vi "Lab Panel V6.00.vi"() -> ()   [LabVIEW 2017] (continued)
                        n3252 = Unbundle By Name(w5931) -> ("1 (TL) cal"=w5926:dbl, "1 (TN) cal"=w5925:dbl, "2 (TL) cal"=w5924:dbl, "2 (TN) cal"=w5923:dbl)  [unwired: 6 out]
                        n3253 = local write "TEMP LA03"(w5920) -> ()
                        n3254 = Multiply(x=w5919, y=w5926) -> (x*y=w5912:dbl)
                        n3255 = Multiply(x=w5918, y=w5925) -> (x*y=w5911:dbl)
                        n3256 = Multiply(x=w5917, y=w5924) -> (x*y=w5908:dbl)
                        n3257 = Multiply(x=w5916, y=w5923) -> (x*y=w5907:dbl)
                        n3258 = case shown="True" w5903 {
                          tunnel: w5908 -> [w5933 w5938]
                          tunnel: w5913 -> [_ w5936]
                          tunnel: [w5933 w5937] -> w5906
                          tunnel: w5907 -> [w5932 w5935]
                          tunnel: [w5932 w5934] -> w5905
                          frame False {
                          }
                          frame True {
                            n3259 = Multiply(x=w5936, y=w5935) -> (x*y=w5934:dbl)
                            n3260 = Multiply(x=w5936, y=w5938) -> (x*y=w5937:dbl)
                          }
                        }
                        n3261 = case shown="True" w5904 {
                          tunnel: w5912 -> [w5940 w5945]
                          tunnel: w5913 -> [_ w5943]
                          tunnel: [w5940 w5944] -> w5910
                          tunnel: w5911 -> [w5939 w5942]
                          tunnel: [w5939 w5941] -> w5909
                          frame False {
                          }
                          frame True {
                            n3262 = Multiply(x=w5943, y=w5942) -> (x*y=w5941:dbl)
                            n3263 = Multiply(x=w5943, y=w5945) -> (x*y=w5944:dbl)
                          }
                        }
                        n3264 = local read "SIG LAB03-2"() -> (w5928:T2)
                        n3265 = local read "SIG LAB03-1"() -> (w5930:T2)
                        n3266 = Bundle By Name(cluster=w5928, "Tmp Live"=w5906, "Tmp Neut"=w5905) -> (w5927:T2)
                        n3267 = Bundle By Name(cluster=w5930, "Tmp Live"=w5910, "Tmp Neut"=w5909) -> (w5929:T2)
                        n3268 = local write "SIG LAB03-2"(w5927) -> ()
                        n3269 = local write "SIG LAB03-1"(w5929) -> ()
                      }
                      frame #4 {
                        n3270 = case shown="False" w5960 {
                          tunnel: [w5991 w5992] -> w5976
                          tunnel: w5959 -> [_ w5992]
                          frame False {
                            n3271 = local read "CAL LAB04"() -> (w5991:T15)
                          }
                          frame True {
                          }
                        }
                        n3272 = local read "LAB04 TEMP"() -> (w5966:T13)
                        n3273 = local read "TEMP LA04"() -> (w5967:T10)
                        n3274 = call "sub vi - temperature delay v4.vi"("2-run"=w5948, "1-run"=w5949, "temp values IN"=w5967, "temp signals"=w5966) -> ("T2-N"=w5961:dbl, "T2-L"=w5962:dbl, "T1-N"=w5963:dbl, "T1-L"=w5964:dbl, "temp values OUT"=w5965:T47)  [unwired: 3 in]
                        n3275 = Unbundle By Name(w5976) -> ("1 (TL) cal"=w5971:dbl, "1 (TN) cal"=w5970:dbl, "2 (TL) cal"=w5969:dbl, "2 (TN) cal"=w5968:dbl)  [unwired: 6 out]
                        n3276 = local write "TEMP LA04"(w5965) -> ()
                        n3277 = Multiply(x=w5964, y=w5971) -> (x*y=w5957:dbl)
                        n3278 = Multiply(x=w5963, y=w5970) -> (x*y=w5956:dbl)
                        n3279 = Multiply(x=w5962, y=w5969) -> (x*y=w5953:dbl)
                        n3280 = Multiply(x=w5961, y=w5968) -> (x*y=w5952:dbl)
                        n3281 = case shown="True" w5948 {
                          tunnel: w5953 -> [w5978 w5983]
                          tunnel: w5958 -> [_ w5981]
                          tunnel: [w5978 w5982] -> w5951
                          tunnel: w5952 -> [w5977 w5980]
                          tunnel: [w5977 w5979] -> w5950
                          frame False {
                          }
                          frame True {
                            n3282 = Multiply(x=w5981, y=w5980) -> (x*y=w5979:dbl)
                            n3283 = Multiply(x=w5981, y=w5983) -> (x*y=w5982:dbl)
                          }
                        }
                        n3284 = case shown="True" w5949 {
                          tunnel: w5957 -> [w5985 w5990]
                          tunnel: w5958 -> [_ w5988]
                          tunnel: [w5985 w5989] -> w5955
                          tunnel: w5956 -> [w5984 w5987]
                          tunnel: [w5984 w5986] -> w5954
                          frame False {
                          }
                          frame True {
                            n3285 = Multiply(x=w5988, y=w5987) -> (x*y=w5986:dbl)
                            n3286 = Multiply(x=w5988, y=w5990) -> (x*y=w5989:dbl)
                          }
                        }
                        n3287 = local read "SIG LAB04-2"() -> (w5973:T2)
                        n3288 = local read "SIG LAB04-1"() -> (w5975:T2)
                        n3289 = Bundle By Name(cluster=w5973, "Tmp Live"=w5951, "Tmp Neut"=w5950) -> (w5972:T2)
                        n3290 = Bundle By Name(cluster=w5975, "Tmp Live"=w5955, "Tmp Neut"=w5954) -> (w5974:T2)
                        n3291 = local write "SIG LAB04-2"(w5972) -> ()
                        n3292 = local write "SIG LAB04-1"(w5974) -> ()
                      }
                      frame #5 {
                        n3293 = case shown="False" w6005 {
                          tunnel: [w6036 w6037] -> w6021
                          tunnel: w6004 -> [_ w6037]
                          frame False {
                            n3294 = local read "CAL LAB05"() -> (w6036:T15)
                          }
                          frame True {
                          }
                        }
                        n3295 = local read "LAB05 TEMP"() -> (w6011:T13)
                        n3296 = local read "TEMP LA05"() -> (w6012:T10)
                        n3297 = call "sub vi - temperature delay v4.vi"("2-run"=w5993, "1-run"=w5994, "temp values IN"=w6012, "temp signals"=w6011) -> ("T2-N"=w6007:dbl, "T2-L"=w6008:dbl, "T1-N"=w6009:dbl, "T1-L"=w6010:dbl, "temp values OUT"=w6006:T47)  [unwired: 3 in]
                        n3298 = local write "TEMP LA05"(w6006) -> ()
                        n3299 = Unbundle By Name(w6021) -> ("1 (TL) cal"=w6013:dbl, "1 (TN) cal"=w6016:dbl, "2 (TL) cal"=w6015:dbl, "2 (TN) cal"=w6014:dbl)  [unwired: 6 out]
                        n3300 = Multiply(x=w6010, y=w6013) -> (x*y=w6002:dbl)
                        n3301 = Multiply(x=w6009, y=w6016) -> (x*y=w6001:dbl)
                        n3302 = Multiply(x=w6008, y=w6015) -> (x*y=w5998:dbl)
                        n3303 = Multiply(x=w6007, y=w6014) -> (x*y=w5997:dbl)
                        n3304 = case shown="True" w5993 {
                          tunnel: w5998 -> [w6023 w6028]
                          tunnel: w6003 -> [_ w6026]
                          tunnel: [w6023 w6027] -> w5996
                          tunnel: w5997 -> [w6022 w6025]
                          tunnel: [w6022 w6024] -> w5995
                          frame False {
                          }
                          frame True {
                            n3305 = Multiply(x=w6026, y=w6025) -> (x*y=w6024:dbl)
                            n3306 = Multiply(x=w6026, y=w6028) -> (x*y=w6027:dbl)
                          }
                        }
                        n3307 = case shown="True" w5994 {
                          tunnel: w6002 -> [w6030 w6035]
                          tunnel: w6003 -> [_ w6033]
                          tunnel: [w6030 w6034] -> w6000
                          tunnel: w6001 -> [w6029 w6032]
                          tunnel: [w6029 w6031] -> w5999
                          frame False {
                          }
                          frame True {
                            n3308 = Multiply(x=w6033, y=w6032) -> (x*y=w6031:dbl)
                            n3309 = Multiply(x=w6033, y=w6035) -> (x*y=w6034:dbl)
                          }
                        }
                        n3310 = local read "SIG LAB05-1"() -> (w6020:T2)
                        n3311 = Bundle By Name(cluster=w6020, "Tmp Live"=w6000, "Tmp Neut"=w5999) -> (w6019:T2)
                        n3312 = local read "SIG LAB05-2"() -> (w6018:T2)
                        n3313 = Bundle By Name(cluster=w6018, "Tmp Live"=w5996, "Tmp Neut"=w5995) -> (w6017:T2)
                        n3314 = local write "SIG LAB05-1"(w6019) -> ()
                        n3315 = local write "SIG LAB05-2"(w6017) -> ()
                      }
                      frame #6 {
                        w6138 = 150.0
                        # "check for thermocouple error, output >150 deg??"
                        n3316 = local read "SIG LAB01-2"() -> (w6147:T2)
                        n3317 = local read "SIG LAB01-1"() -> (w6148:T2)
                        n3318 = local read "SIG LAB04-1"() -> (w6141:T2)
                        n3319 = local read "SIG LAB04-2"() -> (w6142:T2)
                        n3320 = Unbundle By Name(w6148) -> ("Tmp Live"=w6076:dbl, "Tmp Neut"=w6074:dbl)
                        n3321 = Unbundle(w6142) -> ("Tmp Live"=w6052:dbl, "Tmp Neut"=w6051:dbl)  [unwired: 3 out]
                        n3322 = Unbundle(w6147) -> ("Tmp Live"=w6073:dbl, "Tmp Neut"=w6071:dbl)  [unwired: 3 out]
                        n3323 = Unbundle(w6141) -> ("Tmp Live"=w6053:dbl, "Tmp Neut"=w6046:dbl)  [unwired: 3 out]
                        n3324 = Absolute Value(x=w6053) -> (abs(x)=w6047:dbl)
                        n3325 = Absolute Value(x=w6046) -> (abs(x)=w6048:dbl)
                        n3326 = Absolute Value(x=w6052) -> (abs(x)=w6050:dbl)
                        n3327 = Absolute Value(x=w6051) -> (abs(x)=w6049:dbl)
                        n3328 = Absolute Value(x=w6073) -> (abs(x)=w6072:dbl)
                        n3329 = Absolute Value(x=w6071) -> (abs(x)=w6070:dbl)
                        n3330 = Absolute Value(x=w6074) -> (abs(x)=w6075:dbl)
                        n3331 = Absolute Value(x=w6076) -> (abs(x)=w6077:dbl)
                        n3332 = Greater?(x=w6049, y=w6138) -> (0:w6114:bool)
                        "LA04-2 (TN)" <- w6114
                        n3333 = Greater?(x=w6070, y=w6138) -> (0:w6126:bool)
                        "LA01-2 (TN)" <- w6126
                        n3334 = Greater?(x=w6050, y=w6138) -> (0:w6115:bool)
                        "LA04-2 (TL)" <- w6115
                        n3335 = Greater?(x=w6072, y=w6138) -> (0:w6127:bool)
                        "LA01-2 (TL)" <- w6127
                        n3336 = Greater?(x=w6048, y=w6138) -> (0:w6116:bool)
                        "LA04-1 (TN)" <- w6116
                        n3337 = Greater?(x=w6075, y=w6138) -> (0:w6137:bool)
                        "LA01-1 (TN)" <- w6137
                        n3338 = Greater?(x=w6047, y=w6138) -> (0:w6117:bool)
                        "LA04-1 (TL)" <- w6117
                        n3339 = Greater?(x=w6077, y=w6138) -> (0:w6136:bool)
                        "LA01-1 (TL)" <- w6136
                        n3340 = Or(x=w6137, y=w6136) -> (x .or. y?=w6135:bool)
                        n3341 = Or(x=w6114, y=w6115) -> (x .or. y?=w6125:bool)
                        n3342 = Or(x=w6127, y=w6126) -> (x .or. y?=w6131:bool)
                        n3343 = Or(x=w6116, y=w6117) -> (x .or. y?=w6121:bool)
                        n3344 = Select(t=u32 16711680, s=w6135, f=u32 13816530) -> (s? t:f=w6132:u32)
                        n3345 = Select(t=u32 16711680, s=w6125, f=u32 13816530) -> (s? t:f=w6122:u32)
                        n3346 = Select(t=u32 16711680, s=w6131, f=u32 13816530) -> (s? t:f=w6128:u32)
                        n3347 = Select(t=u32 16711680, s=w6121, f=u32 13816530) -> (s? t:f=w6118:u32)
                        n3348 = property on="SIG LAB01-1" class="Clust (strict)"("Color"=w6132) -> ()  [unwired: 2 in, 2 out]
                        n3349 = property on="SIG LAB01-2" class="Clust (strict)"("Color"=w6128) -> ()  [unwired: 2 in, 2 out]
                        n3350 = property on="SIG LAB04-2" class="Clust (strict)"("Color"=w6122) -> ()  [unwired: 2 in, 2 out]
                        n3351 = property on="SIG LAB04-1" class="Clust (strict)"("Color"=w6118) -> ()  [unwired: 2 in, 2 out]
                        n3352 = local read "SIG LAB02-1"() -> (w6145:T2)
                        n3353 = local read "SIG LAB02-2"() -> (w6146:T2)
                        n3354 = local read "SIG LAB05-2"() -> (w6139:T2)
                        n3355 = local read "SIG LAB05-1"() -> (w6140:T2)
                        n3356 = Unbundle(w6146) -> ("Tmp Live"=w6065:dbl, "Tmp Neut"=w6063:dbl)  [unwired: 3 out]
                        n3357 = Unbundle(w6145) -> ("Tmp Live"=w6069:dbl, "Tmp Neut"=w6068:dbl)  [unwired: 3 out]
                        n3358 = Unbundle(w6139) -> ("Tmp Live"=w6041:dbl, "Tmp Neut"=w6039:dbl)  [unwired: 3 out]
                        n3359 = Unbundle(w6140) -> ("Tmp Live"=w6045:dbl, "Tmp Neut"=w6043:dbl)  [unwired: 3 out]
                        n3360 = Absolute Value(x=w6065) -> (abs(x)=w6064:dbl)
                        n3361 = Absolute Value(x=w6063) -> (abs(x)=w6062:dbl)
                        n3362 = Absolute Value(x=w6068) -> (abs(x)=w6066:dbl)
                        n3363 = Absolute Value(x=w6069) -> (abs(x)=w6067:dbl)
                        n3364 = Absolute Value(x=w6041) -> (abs(x)=w6040:dbl)
                        n3365 = Absolute Value(x=w6039) -> (abs(x)=w6038:dbl)
                        n3366 = Absolute Value(x=w6045) -> (abs(x)=w6044:dbl)
                        n3367 = Absolute Value(x=w6043) -> (abs(x)=w6042:dbl)
                        n3368 = Greater?(x=w6062, y=w6138) -> (0:w6090:bool)
                        "LA02-2 (TN)" <- w6090
                        n3369 = Greater?(x=w6064, y=w6138) -> (0:w6091:bool)
                        "LA02-2 (TL)" <- w6091
                        n3370 = Greater?(x=w6066, y=w6138) -> (0:w6093:bool)
                        "LA02-1 (TN)" <- w6093
                        n3371 = Greater?(x=w6067, y=w6138) -> (0:w6092:bool)
                        "LA02-1 (TL)" <- w6092
                        n3372 = Greater?(x=w6038, y=w6138) -> (0:w6102:bool)
                        "LA05-2 (TN)" <- w6102
                        n3373 = Greater?(x=w6040, y=w6138) -> (0:w6103:bool)
                        "LA05-2 (TL)" <- w6103
                        n3374 = Greater?(x=w6042, y=w6138) -> (0:w6104:bool)
                        "LA05-1 (TN)" <- w6104
                        n3375 = Greater?(x=w6044, y=w6138) -> (0:w6105:bool)
                        "LA05-1 (TL)" <- w6105
                        n3376 = Or(x=w6093, y=w6092) -> (x .or. y?=w6101:bool)
                        n3377 = Or(x=w6091, y=w6090) -> (x .or. y?=w6097:bool)
                        n3378 = Or(x=w6105, y=w6104) -> (x .or. y?=w6113:bool)
                        n3379 = Or(x=w6103, y=w6102) -> (x .or. y?=w6109:bool)
                        n3380 = Select(t=u32 16711680, s=w6101, f=u32 13816530) -> (s? t:f=w6098:u32)
                        n3381 = Select(t=u32 16711680, s=w6097, f=u32 13816530) -> (s? t:f=w6094:u32)
                        n3382 = Select(t=u32 16711680, s=w6113, f=u32 13816530) -> (s? t:f=w6110:u32)
                        n3383 = local read "SIG LAB03-1"() -> (w6143:T2)
                        n3384 = Select(t=u32 16711680, s=w6109, f=u32 13816530) -> (s? t:f=w6106:u32)
                        n3385 = property on="SIG LAB02-1" class="Clust (strict)"("Color"=w6098) -> ()  [unwired: 2 in, 2 out]
                        n3386 = property on="SIG LAB02-2" class="Clust (strict)"("Color"=w6094) -> ()  [unwired: 2 in, 2 out]
                        n3387 = local read "SIG LAB03-2"() -> (w6144:T2)
                        n3388 = property on="SIG LAB05-1" class="Clust (strict)"("Color"=w6110) -> ()  [unwired: 2 in, 2 out]
                        n3389 = property on="SIG LAB05-2" class="Clust (strict)"("Color"=w6106) -> ()  [unwired: 2 in, 2 out]
                        n3390 = Unbundle(w6144) -> ("Tmp Live"=w6057:dbl, "Tmp Neut"=w6055:dbl)  [unwired: 3 out]
                        n3391 = Unbundle(w6143) -> ("Tmp Live"=w6061:dbl, "Tmp Neut"=w6059:dbl)  [unwired: 3 out]
                        n3392 = Absolute Value(x=w6057) -> (abs(x)=w6056:dbl)
                        n3393 = Absolute Value(x=w6055) -> (abs(x)=w6054:dbl)
                        n3394 = Absolute Value(x=w6061) -> (abs(x)=w6060:dbl)
                        n3395 = Absolute Value(x=w6059) -> (abs(x)=w6058:dbl)
                        n3396 = Greater?(x=w6054, y=w6138) -> (0:w6078:bool)
                        "LA03-2 (TN)" <- w6078
                        n3397 = Greater?(x=w6056, y=w6138) -> (0:w6079:bool)
                        "LA03-2 (TL)" <- w6079
                        n3398 = Greater?(x=w6058, y=w6138) -> (0:w6081:bool)
                        "LA03-1 (TN)" <- w6081
                        n3399 = Greater?(x=w6060, y=w6138) -> (0:w6080:bool)
                        "LA03-1 (TL)" <- w6080
                        n3400 = Or(x=w6081, y=w6080) -> (x .or. y?=w6089:bool)
                        n3401 = Or(x=w6079, y=w6078) -> (x .or. y?=w6085:bool)
                        n3402 = Select(t=u32 16711680, s=w6089, f=u32 13816530) -> (s? t:f=w6086:u32)
                        n3403 = Select(t=u32 16711680, s=w6085, f=u32 13816530) -> (s? t:f=w6082:u32)
                        n3404 = property on="SIG LAB03-1" class="Clust (strict)"("Color"=w6086) -> ()  [unwired: 2 in, 2 out]
                        n3405 = property on="SIG LAB03-2" class="Clust (strict)"("Color"=w6082) -> ()  [unwired: 2 in, 2 out]
                      }
                    }
                  }
                }
              }
            }
          }
          frame #22 {
            # "SAVE ON AMPS VALUES FOR REPORT FILE"
            # "write data to display panel"
            n3406 = global write "Global display 1.vi" "TEST 5-2"(w6184) -> ()
            n3407 = global write "Global display 1.vi" "TEST 4-2"(w6186) -> ()
            n3408 = global write "Global display 1.vi" "TEST 1-2"(w6192) -> ()
            n3409 = global write "Global display 1.vi" "TEST 3-1"(w6189) -> ()
            n3410 = global write "Global display 1.vi" "TEST 5-1"(w6185) -> ()
            n3411 = global write "Global display 1.vi" "TEST 1-1"(w6193) -> ()
            n3412 = global write "Global display 1.vi" "TEST 3-2"(w6188) -> ()
            n3413 = global write "Global display 1.vi" "TEST 4-1"(w6187) -> ()
            n3414 = global write "Global display 1.vi" "TEST 2-2"(w6190) -> ()
            n3415 = global write "Global display 1.vi" "TEST 2-1"(w6191) -> ()
            n3416 = global read "Global display 3.vi" "log 1-1"() -> (→"LOG LAB01-1":string)
            n3417 = global read "Global display 3.vi" "log 3-1"() -> (→"LOG LAB03-1":string)
            n3418 = global read "Global display 3.vi" "log 1-2"() -> (→"LOG LAB01-2":string)
            n3419 = property on="Tab Control 2" class="TabCtl (strict)"() -> ("Pages"=w6183:refnum<vi>[])  [unwired: 2 in, 2 out]
            n3420 = global read "Global display 3.vi" "log 2-1"() -> (→"LOG LAB02-1":string)
            n3421 = global read "Global display 3.vi" "log 2-2"() -> (→"LOG LAB02-2":string)
            n3422 = global read "Global display 3.vi" "log 4-2"() -> (→"LOG LAB04-2":string)
            n3423 = global read "Global display 3.vi" "log 5-2"() -> (→"LOG LAB05-2":string)
            n3424 = global read "Global display 3.vi" "log 5-1"() -> (→"LOG LAB05-1":string)
            n3425 = global read "Global display 3.vi" "log 4-1"() -> (→"LOG LAB04-1":string)
            n3426 = global read "Global display 3.vi" "log 3-2"() -> (→"LOG LAB03-2":string)
            n3427 = Index Array(array=w6183, index=8) -> (element=w6181:refnum<vi>)
            n3428 = property class="Page"(reference=w6181) -> ("PageVis"=w6180:bool)  [unwired: 1 in, 2 out]
            n3429 = local read "DISP LAB03-1"() -> (w6219:T4)
            n3430 = local read "DISP LAB04-2"() -> (w6216:T4)
            n3431 = local read "DISP LAB05-1"() -> (w6215:T4)
            n3432 = local read "DISP LAB01-2"() -> (w6222:T4)
            n3433 = local read "DISP LAB02-1"() -> (w6221:T4)
            n3434 = local read "DISP LAB02-2"() -> (w6220:T4)
            n3435 = local read "DISP LAB04-1"() -> (w6217:T4)
            n3436 = local read "DISP LAB05-2"() -> (w6214:T4)
            n3437 = local read "DISP LAB01-1"() -> (w6223:T4)
            n3438 = local read "DISP LAB03-2"() -> (w6218:T4)
            n3439 = global write "Global display 3.vi" "admin"(w6180) -> ()
            n3440 = local read "O/I  LAB05-2"() -> (w6234:bool)
            n3441 = local read "O/I  LAB05-1"() -> (w6235:bool)
            n3442 = local read "O/I  LAB03-2"() -> (w6238:bool)
            n3443 = local read "O/I  LAB04-2"() -> (w6236:bool)
            n3444 = local read "O/I  LAB04-1"() -> (w6237:bool)
            n3445 = local read "O/I  LAB03-1"() -> (w6239:bool)
            n3446 = local read "O/I  LAB01-2"() -> (w6242:bool)
            n3447 = local read "O/I  LAB01-1"() -> (w6243:bool)
            n3448 = local read "O/I  LAB02-1"() -> (w6241:bool)
            n3449 = local read "O/I  LAB02-2"() -> (w6240:bool)
            n3450 = global write "Global display 1.vi" "5-2 O/F"(w6234) -> ()
            n3451 = global write "Global display 1.vi" "5-1 O/F"(w6235) -> ()
            n3452 = global write "Global display 1.vi" "4-1 O/F"(w6237) -> ()
            n3453 = global write "Global display 1.vi" "4-2 O/F"(w6236) -> ()
            n3454 = global write "Global display 2.vi" "DISP LAB02-1"(w6221) -> ()
            n3455 = global write "Global display 2.vi" "DISP LAB02-2"(w6220) -> ()
            n3456 = global write "Global display 2.vi" "DISP LAB05-1"(w6215) -> ()
            n3457 = global write "Global display 2.vi" "DISP LAB05-2"(w6214) -> ()
            n3458 = global write "Global display 1.vi" "3-2 O/F"(w6238) -> ()
            n3459 = global write "Global display 2.vi" "DISP LAB01-2"(w6222) -> ()
            n3460 = global write "Global display 2.vi" "DISP LAB04-2"(w6216) -> ()
            n3461 = global write "Global display 2.vi" "DISP LAB01-1"(w6223) -> ()
            n3462 = global write "Global display 2.vi" "DISP LAB03-1"(w6219) -> ()
            n3463 = global write "Global display 1.vi" "3-1 O/F"(w6239) -> ()
            n3464 = global write "Global display 2.vi" "DISP LAB04-1"(w6217) -> ()
            n3465 = global write "Global display 1.vi" "2-2 O/F"(w6240) -> ()
            n3466 = global write "Global display 2.vi" "DISP LAB03-2"(w6218) -> ()
            n3467 = global write "Global display 1.vi" "2-1 O/F"(w6241) -> ()
            n3468 = global write "Global display 1.vi" "1-2 O/F"(w6242) -> ()
            n3469 = global write "Global display 1.vi" "1-1 O/F"(w6243) -> ()
            n3470 = local read "run lab05-2"() -> (w6224:bool)
            n3471 = local read "run lab04-1"() -> (w6227:bool)
            n3472 = local read "run lab04-2"() -> (w6226:bool)
            n3473 = local read "run lab05-1"() -> (w6225:bool)
            n3474 = local read "TEMP START LAB02-2"() -> (w6166:cluster{"TL":dbl, "TN":dbl})
            n3475 = local read "TEMP START LAB01-2"() -> (w6168:cluster{"TL":dbl, "TN":dbl})
            n3476 = local read "TEMP START LAB02-1"() -> (w6167:cluster{"TL":dbl, "TN":dbl})
            n3477 = local read "TEMP START LAB04-1"() -> (w6163:cluster{"TL":dbl, "TN":dbl})
            n3478 = local read "TEMP START LAB04-2"() -> (w6162:cluster{"TL":dbl, "TN":dbl})
            n3479 = local read "run lab03-2"() -> (w6228:bool)
            n3480 = local read "TEMP START LAB01-1"() -> (w6169:cluster{"TL":dbl, "TN":dbl})
            n3481 = local read "TEMP START LAB05-2"() -> (w6160:cluster{"TL":dbl, "TN":dbl})
            n3482 = local read "TEMP START LAB05-1"() -> (w6161:cluster{"TL":dbl, "TN":dbl})
            n3483 = local read "run lab02-1"() -> (w6231:bool)
            n3484 = local read "run lab03-1"() -> (w6229:bool)
            n3485 = local read "TEMP START LAB03-2"() -> (w6164:cluster{"TL":dbl, "TN":dbl})
            n3486 = local read "run lab01-2"() -> (w6232:bool)
            n3487 = local read "run lab02-2"() -> (w6230:bool)
            n3488 = local read "TEMP START LAB03-1"() -> (w6165:cluster{"TL":dbl, "TN":dbl})
            n3489 = local read "run lab01-1"() -> (w6233:bool)
            n3490 = global write "Global display 1.vi" "5-2 R/S"(w6224) -> ()
            n3491 = global write "Global display 1.vi" "5-1 R/S"(w6225) -> ()
            n3492 = global write "Global display 1.vi" "4-2 R/S"(w6226) -> ()
            n3493 = global write "Global display 1.vi" "4-1 R/S"(w6227) -> ()
            n3494 = global write "Global display 1.vi" "3-2 R/S"(w6228) -> ()
            n3495 = global write "Global display 1.vi" "1-2 R/S"(w6232) -> ()
            n3496 = global write "Global display 1.vi" "2-1 R/S"(w6231) -> ()
            n3497 = global write "Global display 1.vi" "3-1 R/S"(w6229) -> ()
            n3498 = global write "Global display 1.vi" "2-2 R/S"(w6230) -> ()
            n3499 = global write "Global display 1.vi" "1-1 R/S"(w6233) -> ()
            n3500 = local read "SET LAB05-2"() -> (w6204:T5)
            n3501 = local read "SET LAB05-1"() -> (w6205:T5)
            n3502 = local read "SET LAB04-1"() -> (w6207:T5)
            n3503 = local read "SET LAB04-2"() -> (w6206:T5)
            n3504 = local read "SET LAB01-1"() -> (w6213:T6)
            n3505 = local read "SET LAB03-1"() -> (w6209:T5)
            n3506 = local read "SET LAB03-2"() -> (w6208:T5)
            n3507 = local read "SET LAB02-2"() -> (w6210:T5)
            n3508 = local read "SET LAB01-2"() -> (w6212:T5)
            n3509 = local read "SET LAB02-1"() -> (w6211:T5)
            n3510 = global write "Global display 3.vi" "TEMP ST 05-2"(w6160) -> ()
            n3511 = global write "Global display 3.vi" "TEMP ST 05-1"(w6161) -> ()
            n3512 = global write "Global display 3.vi" "TEMP ST 03-2"(w6164) -> ()
            n3513 = global write "Global display 3.vi" "TEMP ST 04-2"(w6162) -> ()
            n3514 = global write "Global display 3.vi" "TEMP ST 01-1"(w6169) -> ()
            n3515 = global write "Global display 3.vi" "TEMP ST 01-2"(w6168) -> ()
            n3516 = global write "Global display 3.vi" "TEMP ST 04-1"(w6163) -> ()
            n3517 = global write "Global display 3.vi" "TEMP ST 02-1"(w6167) -> ()
            n3518 = global write "Global display 3.vi" "TEMP ST 02-2"(w6166) -> ()
            n3519 = global write "Global display 3.vi" "TEMP ST 03-1"(w6165) -> ()
            n3520 = global write "Global display 2.vi" "SET LAB05-2"(w6204) -> ()
            n3521 = global write "Global display 2.vi" "SET LAB05-1"(w6205) -> ()
            n3522 = global write "Global display 2.vi" "SET LAB04-1"(w6207) -> ()
            n3523 = global write "Global display 2.vi" "SET LAB01-1"(w6213) -> ()
            n3524 = global write "Global display 2.vi" "SET LAB04-2"(w6206) -> ()
            n3525 = global write "Global display 2.vi" "SET LAB03-2"(w6208) -> ()
            n3526 = global write "Global display 2.vi" "SET LAB02-2"(w6210) -> ()
            n3527 = global write "Global display 2.vi" "SET LAB03-1"(w6209) -> ()
            n3528 = global write "Global display 2.vi" "SET LAB01-2"(w6212) -> ()
            n3529 = global write "Global display 2.vi" "SET LAB02-1"(w6211) -> ()
            n3530 = local read "TEMP RISE LAB05-1"() -> (w6151:cluster{"TL":dbl, "TN":dbl})
            n3531 = local read "TEMP RISE LAB05-2"() -> (w6150:cluster{"TL":dbl, "TN":dbl})
            n3532 = local read "TEMP RISE LAB04-2"() -> (w6152:cluster{"TL":dbl, "TN":dbl})
            n3533 = local read "TEMP RISE LAB04-1"() -> (w6153:cluster{"TL":dbl, "TN":dbl})
            n3534 = local read "TEMP RISE LAB03-2"() -> (w6154:cluster{"TL":dbl, "TN":dbl})
            n3535 = local read "TEMP RISE LAB03-1"() -> (w6155:cluster{"TL":dbl, "TN":dbl})
            n3536 = local read "TEMP RISE LAB01-2"() -> (w6158:cluster{"TL":dbl, "TN":dbl})
            n3537 = local read "TEMP RISE LAB02-2"() -> (w6156:cluster{"TL":dbl, "TN":dbl})
            n3538 = local read "TEMP RISE LAB01-1"() -> (w6159:cluster{"TL":dbl, "TN":dbl})
            n3539 = local read "TEMP RISE LAB02-1"() -> (w6157:cluster{"TL":dbl, "TN":dbl})
            n3540 = local read "RESULT LAB01-1"() -> (w6203:bool)
            n3541 = local read "RESULT LAB03-2"() -> (w6198:bool)
            n3542 = local read "RESULT LAB04-1"() -> (w6197:bool)
            n3543 = local read "RESULT LAB04-2"() -> (w6196:bool)
            n3544 = local read "RESULT LAB02-2"() -> (w6200:bool)
            n3545 = local read "RESULT LAB01-2"() -> (w6202:bool)
            n3546 = local read "RESULT LAB02-1"() -> (w6201:bool)
            n3547 = local read "RESULT LAB03-1"() -> (w6199:bool)
            n3548 = local read "RESULT LAB05-1"() -> (w6195:bool)
            n3549 = local read "RESULT LAB05-2"() -> (w6194:bool)
            n3550 = local read "Amps Fail level"() -> (w6149:dbl)
            n3551 = stacked-sequence {
              tunnel: w6149 -> [w6245 w6250 w6255 w6260 w6265 w6270 w6275 w6280 w6285 w6290]
              frame #0 {
                n3552 = local read "SIG LAB01-1"() -> (w6247:T2)
                n3553 = Unbundle(w6247) -> ("AMPS"=w6246:dbl)  [unwired: 4 out]
                n3554 = Greater?(x=w6246, y=w6245) -> (0:w6244:bool)
                n3555 = case shown="True" w6244 {
                  frame False {
                  }
                  frame True {
                    n3556 = local read "ON L01-1"() -> (w6248:cluster{"amps":dbl, "volts":dbl, "pf":dbl})
                    n3557 = global write "Global display 2.vi" "ON L01-1"(w6248) -> ()
                  }
                }
              }
              frame #1 {
                n3558 = local read "SIG LAB01-2"() -> (w6252:T2)
                n3559 = Unbundle By Name(w6252) -> ("AMPS"=w6251:dbl)
                n3560 = Greater?(x=w6251, y=w6250) -> (0:w6249:bool)
                n3561 = case shown="True" w6249 {
                  frame False {
                  }
                  frame True {
                    n3562 = local read "ON L01-2"() -> (w6253:cluster{"amps":dbl, "volts":dbl, "pf":dbl})
                    n3563 = global write "Global display 2.vi" "ON L01-2"(w6253) -> ()
                  }
                }
              }
              frame #2 {
                n3564 = local read "SIG LAB02-1"() -> (w6257:T2)
                n3565 = Unbundle(w6257) -> ("AMPS"=w6256:dbl)  [unwired: 4 out]
                n3566 = Greater?(x=w6256, y=w6255) -> (0:w6254:bool)
                n3567 = case shown="True" w6254 {
                  frame False {
                  }
                  frame True {
                    n3568 = local read "ON L02-1"() -> (w6258:cluster{"amps":dbl, "volts":dbl, "pf":dbl})
                    n3569 = global write "Global display 2.vi" "ON L02-1"(w6258) -> ()
                  }
                }
              }
              frame #3 {
                n3570 = local read "SIG LAB02-2"() -> (w6262:T2)
                n3571 = Unbundle(w6262) -> ("AMPS"=w6261:dbl)  [unwired: 4 out]
                n3572 = Greater?(x=w6261, y=w6260) -> (0:w6259:bool)
                n3573 = case shown="True" w6259 {
                  frame False {
                  }
                  frame True {
                    n3574 = local read "ON L02-2"() -> (w6263:cluster{"amps":dbl, "volts":dbl, "pf":dbl})
                    n3575 = global write "Global display 2.vi" "ON L02-2"(w6263) -> ()
                  }
                }
              }
              frame #4 {
                n3576 = local read "SIG LAB03-1"() -> (w6267:T2)
                n3577 = Unbundle(w6267) -> ("AMPS"=w6266:dbl)  [unwired: 4 out]
                n3578 = Greater?(x=w6266, y=w6265) -> (0:w6264:bool)
                n3579 = case shown="True" w6264 {
                  frame False {
                  }
                  frame True {
                    n3580 = local read "ON L03-1"() -> (w6268:cluster{"amps":dbl, "volts":dbl, "pf":dbl})
                    n3581 = global write "Global display 2.vi" "ON L03-1"(w6268) -> ()
                  }
                }
              }
              frame #5 {
                n3582 = local read "SIG LAB03-2"() -> (w6272:T2)
                n3583 = Unbundle(w6272) -> ("AMPS"=w6271:dbl)  [unwired: 4 out]
                n3584 = Greater?(x=w6271, y=w6270) -> (0:w6269:bool)
                n3585 = case shown="True" w6269 {
                  frame False {
                  }
                  frame True {
                    n3586 = local read "ON L03-2"() -> (w6273:cluster{"amps":dbl, "volts":dbl, "pf":dbl})
                    n3587 = global write "Global display 2.vi" "ON L03-2"(w6273) -> ()
                  }
                }
              }
              frame #6 {
                n3588 = local read "SIG LAB04-1"() -> (w6277:T2)
                n3589 = Unbundle(w6277) -> ("AMPS"=w6276:dbl)  [unwired: 4 out]
                n3590 = Greater?(x=w6276, y=w6275) -> (0:w6274:bool)
                n3591 = case shown="True" w6274 {
                  frame False {
                  }
                  frame True {
                    n3592 = local read "ON L04-1"() -> (w6278:cluster{"amps":dbl, "volts":dbl, "pf":dbl})
                    n3593 = global write "Global display 2.vi" "ON L04-1"(w6278) -> ()
                  }
                }
              }
              frame #7 {
                n3594 = local read "SIG LAB04-2"() -> (w6282:T2)
                n3595 = Unbundle(w6282) -> ("AMPS"=w6281:dbl)  [unwired: 4 out]
                n3596 = Greater?(x=w6281, y=w6280) -> (0:w6279:bool)
                n3597 = case shown="True" w6279 {
                  frame False {
                  }
                  frame True {
                    n3598 = local read "ON L04-2"() -> (w6283:cluster{"amps":dbl, "volts":dbl, "pf":dbl})
                    n3599 = global write "Global display 2.vi" "ON L04-2"(w6283) -> ()
                  }
                }
              }
              frame #8 {
                n3600 = local read "SIG LAB05-1"() -> (w6287:T2)
                n3601 = Unbundle(w6287) -> ("AMPS"=w6286:dbl)  [unwired: 4 out]
                n3602 = Greater?(x=w6286, y=w6285) -> (0:w6284:bool)
                n3603 = case shown="True" w6284 {
                  frame False {
                  }
                  frame True {
                    n3604 = local read "ON L05-1"() -> (w6288:cluster{"amps":dbl, "volts":dbl, "pf":dbl})
                    n3605 = global write "Global display 2.vi" "ON L05-1"(w6288) -> ()
                  }
                }
              }
              frame #9 {
                n3606 = local read "SIG LAB05-2"() -> (w6292:T2)
                n3607 = Unbundle(w6292) -> ("AMPS"=w6291:dbl)  [unwired: 4 out]
                n3608 = Greater?(x=w6291, y=w6290) -> (0:w6289:bool)
                n3609 = case shown="True" w6289 {
                  frame False {
                  }
                  frame True {
                    n3610 = local read "ON L05-2"() -> (w6293:cluster{"amps":dbl, "volts":dbl, "pf":dbl})
                    n3611 = global write "Global display 2.vi" "ON L05-2"(w6293) -> ()
                  }
                }
              }
            }
            n3612 = global write "Global display 3.vi" "TEMP RS 05-2"(w6150) -> ()
            n3613 = global write "Global display 3.vi" "TEMP RS 05-1"(w6151) -> ()
            n3614 = global write "Global display 3.vi" "TEMP RS 03-2"(w6154) -> ()
            n3615 = global write "Global display 3.vi" "TEMP RS 02-1"(w6157) -> ()
            n3616 = global write "Global display 3.vi" "TEMP RS 02-2"(w6156) -> ()
            n3617 = global write "Global display 3.vi" "TEMP RS 04-2"(w6152) -> ()
            n3618 = global write "Global display 3.vi" "TEMP RS 01-2"(w6158) -> ()
            n3619 = global write "Global display 3.vi" "TEMP RS 03-1"(w6155) -> ()
            n3620 = global write "Global display 3.vi" "TEMP RS 04-1"(w6153) -> ()
            n3621 = global write "Global display 3.vi" "TEMP RS 01-1"(w6159) -> ()
            n3622 = global write "Global display 2.vi" "RESULT LAB05-1"(w6195) -> ()
            n3623 = global write "Global display 2.vi" "RESULT LAB01-2"(w6202) -> ()
            n3624 = global write "Global display 2.vi" "RESULT LAB03-2"(w6198) -> ()
            n3625 = global write "Global display 2.vi" "RESULT LAB04-1"(w6197) -> ()
            n3626 = global write "Global display 2.vi" "RESULT LAB04-2"(w6196) -> ()
            n3627 = global write "Global display 2.vi" "RESULT LAB05-2"(w6194) -> ()
            n3628 = global write "Global display 2.vi" "RESULT LAB03-1"(w6199) -> ()
            n3629 = global write "Global display 2.vi" "RESULT LAB01-1"(w6203) -> ()
            n3630 = global write "Global display 2.vi" "RESULT LAB02-1"(w6201) -> ()
            n3631 = global write "Global display 2.vi" "RESULT LAB02-2"(w6200) -> ()
          }
          frame #23 {
            # "simulate values"
            n3632 = global write "Global display 4.vi" "LAB deg C"("LAB deg C") -> ()
          }
          frame #24 {
            # "end main and display program"
            n3633 = stacked-sequence {
              seq-local: [_ w6300 _] -> [_ _ w6306]
              tunnel: w6296 -> [w6297 _ _]
              tunnel: w6295 -> [_ _ w6304]
              frame #0 {
                n3634 = case shown="True" w6297 {
                  frame False {
                  }
                  frame True {
                    n3635 = One Button Dialog(message="Excessive number of USB \nresets done, re-start program.") -> ()  [unwired: 1 in, 1 out]
                  }
                }
              }
              frame #1 {
                # "check for reset error"
                n3636 = local read "Simulate"() -> (w6299:bool)
                n3637 = case shown="False" w6299 {
                  tunnel: [w6301 FALSE] -> w6300
                  frame False {
                    n3638 = local read "Reset Error"() -> (w6301:bool)
                    n3639 = case shown="True" w6301 {
                      frame False {
                      }
                      frame True {
                        n3640 = One Button Dialog(message="USB ERROR, program will be stopped.\nClose program, close windows, switch panel off\nand re power panel. If error persists seek help.") -> ()  [unwired: 1 in, 1 out]
                      }
                    }
                  }
                  frame True {
                  }
                }
              }
              frame #2 {
                # "end labview session"
                n3641 = case shown="True" w6304 {
                  frame False {
                  }
                  frame True {
                    n3642 = call "sub vi - AI USB4704 (3)  Close Task v2.vi"() -> ()  [unwired: 16 in]
                  }
                }
                n3643 = Or(x=w6306, y="stop all") -> (x .or. y?=w6305:bool)
                n3644 = case shown="True" w6305 {
                  frame False {
                  }
                  frame True {
                    n3645 = stacked-sequence {
                      frame #0 {
                        n3646 = global write "Global display 1.vi" "stop disp"(TRUE) -> ()
                      }
                      frame #1 {
                        n3647 = call "sub vi - AI USB4704 (3)  Close Task v2.vi"() -> ()  [unwired: 16 in]
                      }
                      frame #2 {
                        n3648 = Quit LabVIEW(quit? (T)=TRUE) -> ()
                      }
                    }
                  }
                }
              }
            }
          }
        }
        n3649 = node-c288() -> ()  [unwired: 1 in, 1 out]
        "loops" <- w361
      }
      n3650 = node-c288(w333) -> ()  [unwired: 1 out]
    }
  }
